vi "TDC_fitLftHistogram.vi"(8 "Error In":errorcluster, 9 "fct in":u64, 10 "Start Parameters":dbl[](array[numeric]), 11 "Fit Type":u16(ring) items=["None", "Exponential", "Double Exponential", "Kohlrausch"]) -> (0 "Error Out":errorcluster, 2 "Fit Parameters":dbl[](array[numeric]), 3 "Iterations":i32)   [LabVIEW 2011]
uses:
  tdcbase.dll
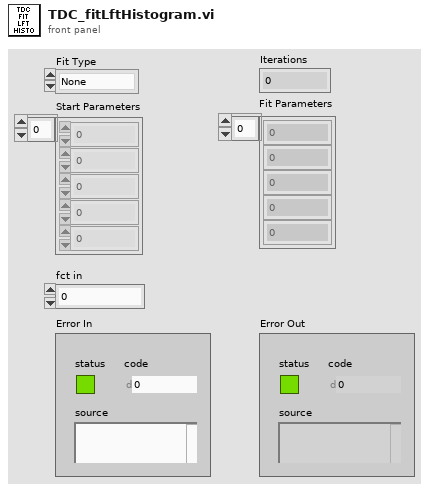
[diagram p1: front panel]
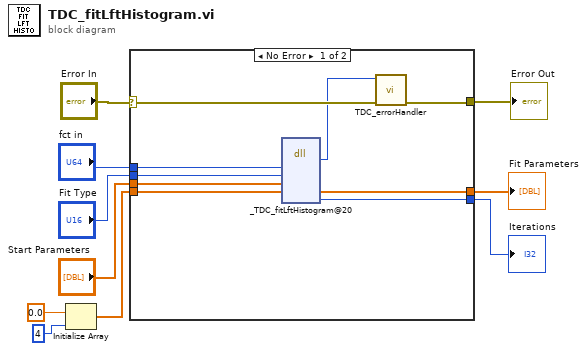
[diagram p0: block diagram]
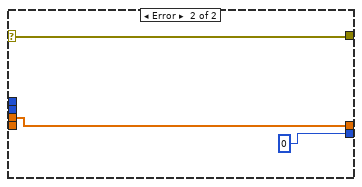
[diagram p2: hidden frame]
diagram:
  n1 = Initialize Array(0.0, 4) -> (w3:dbl[])
  n2 = case shown="No Error" "Error In" {
    selector: "Error In" -> [w18 w22]
    tunnel: [w17 w22] -> w9
    tunnel: "fct in" -> [w19 _]
    tunnel: "Fit Type" -> [w15 _]
    tunnel: "Start Parameters" -> [w14 w21]
    tunnel: w3 -> [w13 _]
    tunnel: [w12 w21] -> w2
    tunnel: [w11 0] -> w1
    frame No Error {
      n3 = dll-call lib="X:/tdcbase.dll" fn="_TDC_fitLftHistogram@20"("fct"=w19, "fitType"=w15, "startParams"=w14, "fitParams"=w13) -> ("return type"=w16:i32, "fitParams"=w12:dbl[], "iterations"=w11:i32)  [unwired: 7 in, 2 out]
      n4 = call "TDC_errorHandler.vi"("Error In"=w18, "TDC Return Code"=w16) -> ("Error Out"=w17:errorcluster)  [unwired: 9 in]
    }
    frame Error {
    }
  }
  "Error Out" <- w9
  "Fit Parameters" <- w2
  "Iterations" <- w1
